vi "VI Tree.vi"   [LabVIEW 2015, in "Lake Shore 372.lvlib"]
doc: "This is the instrument driver for the LakeShore 372 AC Resistance Bridge. The VI Tree displays all the user-callable VIs of the instrument driver in an organized table."
uses:
  <instrlib>/Lake Shore 372/Lake Shore 372.lvlib
panel:
  # "(c) 2015 Advint LLC. ALL RIGHTS RESERVED."
  # "SEE DIAGRAM\nFOR VI TREE."
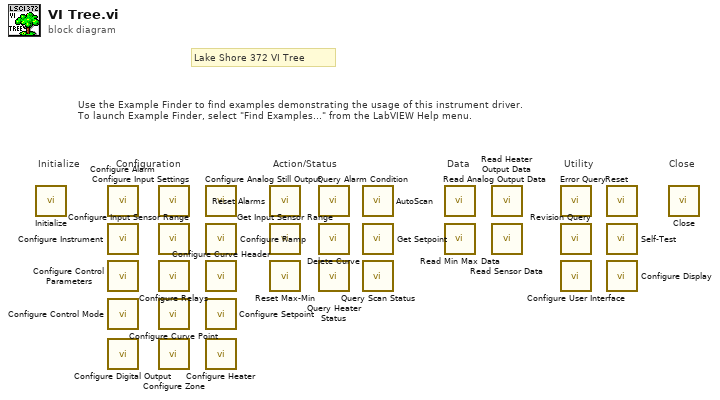
[diagram p0: block diagram]
diagram:
  # "Lake Shore 372 VI Tree"
  # "Initialize"
  # "Close"
  # "Action/Status"
  # "Data"
  # "Utility"
  # "Configuration"
  # "Use the Example Finder to find examples demonstrating the usage of this instrument driver.\nTo launch Example Finder, select \"Find Examples...\" from the LabVIEW Help menu."
  n1 = call <instrlib>:"Initialize.vi"() -> ()  [unwired: 10 in, 2 out]
  n2 = call <instrlib>:"Configure Alarm.vi"() -> ()  [unwired: 14 in, 2 out]
  n3 = call <instrlib>:"Configure Instrument.vi"() -> ()  [unwired: 10 in, 2 out]
  n4 = call <instrlib>:"Configure Control Parameters.vi"() -> ()  [unwired: 14 in, 2 out]
  n5 = call <instrlib>:"Configure Control Mode.vi"() -> ()  [unwired: 14 in, 2 out]
  n6 = call <instrlib>:"Configure Digital Output.vi"() -> ()  [unwired: 10 in, 2 out]
  n7 = call <instrlib>:"Configure Input Settings.vi"() -> ()  [unwired: 18 in, 2 out]
  n8 = call <instrlib>:"Configure Input Sensor Range.vi"() -> ()  [unwired: 18 in, 2 out]
  n9 = call <instrlib>:"Configure Relays.vi"() -> ()  [unwired: 10 in, 2 out]
  n10 = call <instrlib>:"Configure Curve Point.vi"() -> ()  [unwired: 14 in, 2 out]
  n11 = call <instrlib>:"Configure Zone.vi"() -> ()  [unwired: 18 in, 2 out]
  n12 = call <instrlib>:"Configure Analog Still Output.vi"() -> ()  [unwired: 14 in, 2 out]
  n13 = call <instrlib>:"Configure Ramp.vi"() -> ()  [unwired: 10 in, 2 out]
  n14 = call <instrlib>:"Configure Curve Header.vi"() -> ()  [unwired: 14 in, 2 out]
  n15 = call <instrlib>:"Configure Setpoint.vi"() -> ()  [unwired: 10 in, 2 out]
  n16 = call <instrlib>:"Configure Heater.vi"() -> ()  [unwired: 14 in, 2 out]
  n17 = call <instrlib>:"Reset Alarms.vi"() -> ()  [unwired: 10 in, 2 out]
  n18 = call <instrlib>:"Get Input Sensor Range.vi"() -> ()  [unwired: 8 in, 8 out]
  n19 = call <instrlib>:"Reset Max-Min.vi"() -> ()  [unwired: 10 in, 2 out]
  n20 = call <instrlib>:"Query Alarm Condition.vi"() -> ()  [unwired: 8 in, 4 out]
  n21 = call <instrlib>:"Delete Curve.vi"() -> ()  [unwired: 10 in, 2 out]
  n22 = call <instrlib>:"Query Heater Status.vi"() -> ()  [unwired: 9 in, 3 out]
  n23 = call <instrlib>:"AutoScan.vi"() -> ()  [unwired: 10 in, 2 out]
  n24 = call <instrlib>:"Get Setpoint.vi"() -> ()  [unwired: 9 in, 3 out]
  n25 = call <instrlib>:"Query Scan Status.vi"() -> ()  [unwired: 8 in, 4 out]
  n26 = call <instrlib>:"Read Analog Output Data.vi"() -> ()  [unwired: 9 in, 3 out]
  n27 = call <instrlib>:"Read Min Max Data.vi"() -> ()  [unwired: 8 in, 4 out]
  n28 = call <instrlib>:"Read Heater Output Data.vi"() -> ()  [unwired: 9 in, 3 out]
  n29 = call <instrlib>:"Read Sensor Data.vi"() -> ()  [unwired: 6 in, 6 out]
  n30 = call <instrlib>:"Error Query.vi"() -> ()  [unwired: 9 in, 3 out]
  n31 = call <instrlib>:"Revision Query.vi"() -> ()  [unwired: 10 in, 6 out]
  n32 = call <instrlib>:"Configure User Interface.vi"() -> ()  [unwired: 10 in, 2 out]
  n33 = call <instrlib>:"Reset.vi"() -> ()  [unwired: 10 in, 2 out]
  n34 = call <instrlib>:"Self-Test.vi"() -> ()  [unwired: 8 in, 4 out]
  n35 = call <instrlib>:"Configure Display.vi"() -> ()  [unwired: 10 in, 2 out]
  n36 = call <instrlib>:"Close.vi"() -> ()  [unwired: 11 in, 1 out]
